vi "Board Measurement.vi"(4 "index":i32, 5 "Board":T1 items=["Quad DC Board", "Lens 1 (Slot 8) Module", "Lens 2 (Slot 6) Module", "Detector Board", "Quad DC Board with Test Points", "Lens 1 Module with Test Points", "Len 2 Module with Test Points", "", "", "", "", ""], 6 "Expected Reading":dbl, 7 "DAC Channel Name":string) -> (1 "Aborted":bool, 3 "Reading":string)   [LabVIEW 2012]
uses:
  Type/_Board ID.ctl
panel:
  in  "AbortButton":bool
  in  "Actual Reading":string
  in  "Done":bool
  # "Please enter an actual reading for the DAC channel below \n(Use the attached picture to locate test points)"
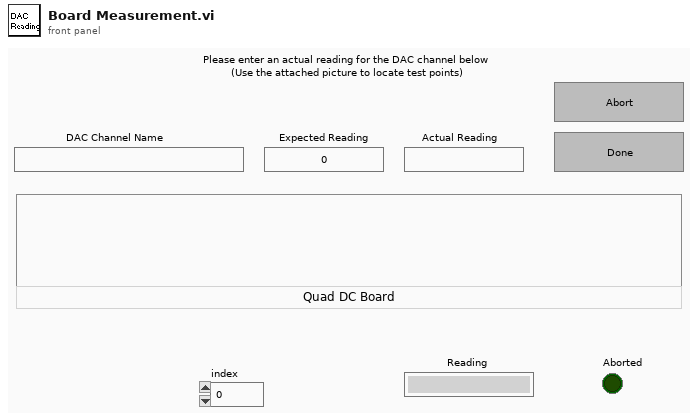
[diagram p1: front panel]
types:
  T1 = typedef "_Board ID.ctl" = u16
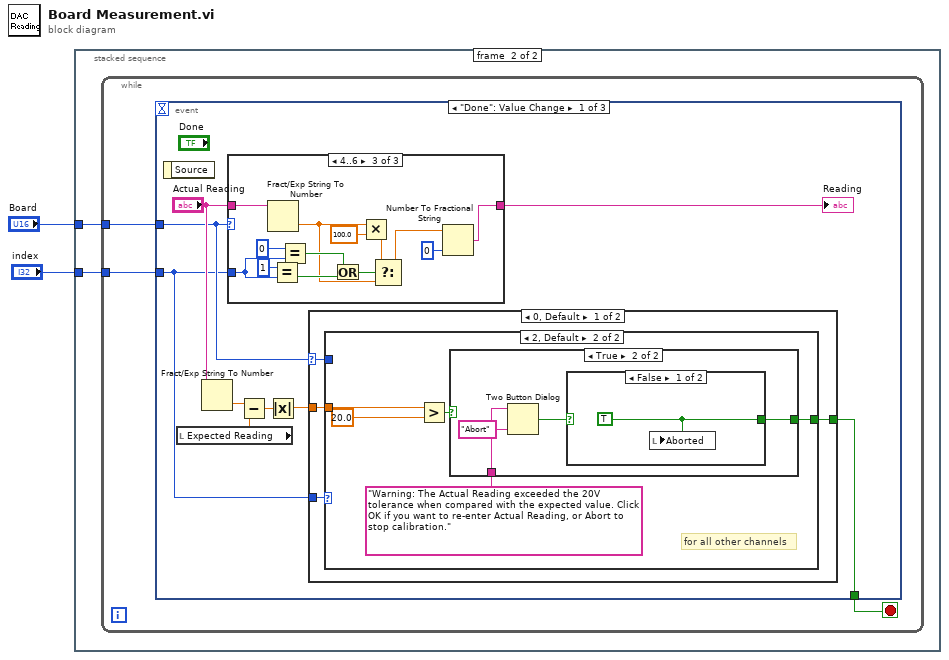
[diagram p0: block diagram]
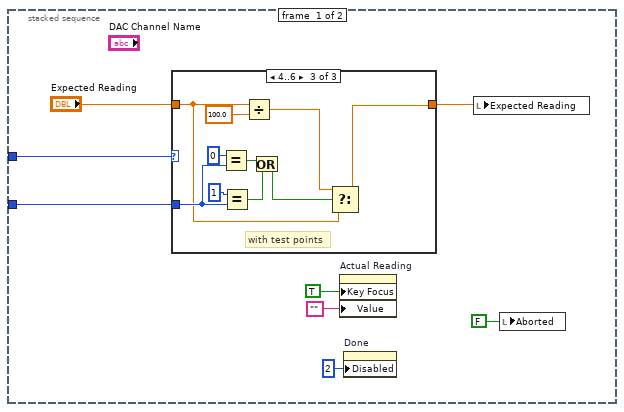
[diagram p2: hidden frame]
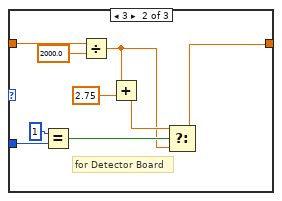
[diagram p4: hidden frame]
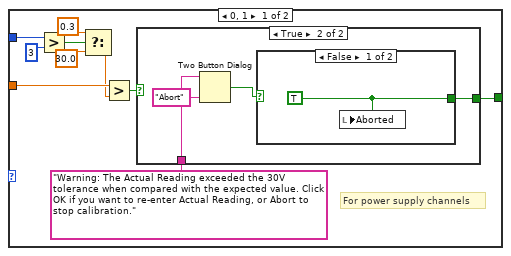
[diagram p5: hidden frame]
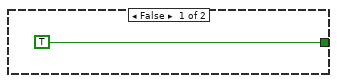
[diagram p6: hidden frame]
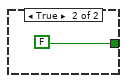
[diagram p7: hidden frame]
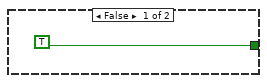
[diagram p8: hidden frame]
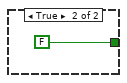
[diagram p9: hidden frame]
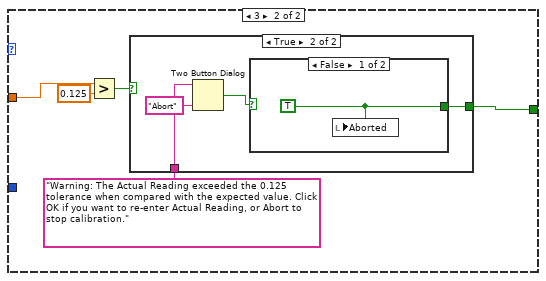
[diagram p10: hidden frame]
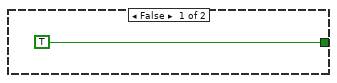
[diagram p11: hidden frame]
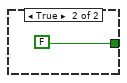
[diagram p12: hidden frame]
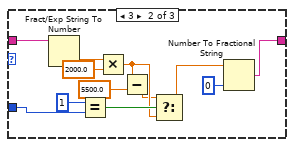
[diagram p14: hidden frame]
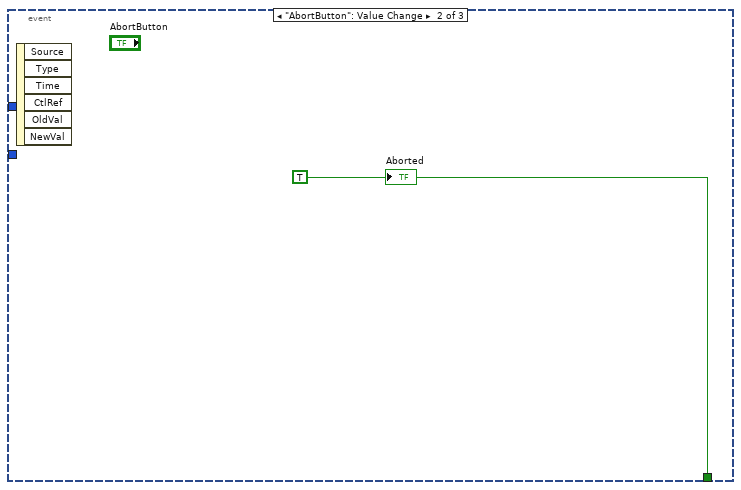
[diagram p15: hidden frame]
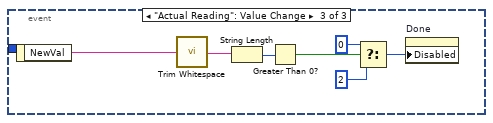
[diagram p16: hidden frame]
diagram:
  n1 = stacked-sequence {
    tunnel: "Board" -> [w7 w32]
    tunnel: "index" -> [w4 w31]
    frame #0 {
      n2 = case shown="4..6" w7 {
        tunnel: "Expected Reading" -> [w11 w20 w21]
        tunnel: [w11 w15 w29] -> w5
        tunnel: w4 -> [_ w18 w26]
        frame 0, Default {
          # "without test points"
        }
        frame 3 {
          # "for Detector Board"
          n3 = Equal?(x=1, y=w18) -> (x = y?=w17:bool)
          n4 = Divide(x=w20, y=2000.0) -> (x/y=w12:dbl)
          n5 = Add(x=w12, y=2.75) -> (x+y=w13:dbl)
          n6 = Select(t=w13, s=w17, f=w12) -> (s? t:f=w15:dbl)
        }
        frame 4..6 {
          # "with test points"
          n7 = Equal?(x=0, y=w26) -> (x = y?=w25:bool)
          n8 = Equal?(x=1, y=w26) -> (x = y?=w24:bool)
          n9 = Divide(x=w21, y=100.0) -> (x/y=w22:dbl)
          n10 = Or(x=w25, y=w24) -> (x .or. y?=w23:bool)
          n11 = Select(t=w22, s=w23, f=w21) -> (s? t:f=w29:dbl)
        }
      }
      n12 = property on="Actual Reading" class="Str"("Key Focus"=TRUE, "Value"="") -> ()  [unwired: 2 in, 2 out]
      n13 = property on="Done" class="Bool"("Disabled"=u8 2) -> ()  [unwired: 2 in, 2 out]
      n14 = local write "Expected Reading"(w5) -> ()
      n15 = local write "Aborted"(FALSE ("Aborted")) -> ()
    }
    frame #1 {
      n16 = while {
        tunnel: w32 -> [w34]
        tunnel: w31 -> [w33]
        stop <- w35 stop-if-true
        n17 = event shown="[0] \"Done\": Value Change" {
          selector: _ -> [_ _ _]
          dyn-events: _ -> [_ _ _]
          timeout: _ -> [_ _ _]
          tunnel: [w38 w116 _] -> w35
          tunnel: w34 -> [w37 _ _]
          tunnel: w33 -> [w36 _ _]
          event "Done": Value Change {
            n18 = event-data() -> ()  [unwired: 2 out]
            n19 = local read "Expected Reading"() -> (w41:dbl)
            n20 = Fract/Exp String To Number(string="Actual Reading") -> (number=w42:dbl)  [unwired: 4 out]
            n21 = case shown="4..6" w37 {
              tunnel: [w90 w98 w112] -> w44
              tunnel: "Actual Reading" -> [w90 w102 w115]
              tunnel: w36 -> [_ w96 w108]
              frame 0, Default {
              }
              frame 3 {
                n22 = Fract/Exp String To Number(string=w102) -> (number=w101:dbl)  [unwired: 4 out]
                n23 = Equal?(x=1, y=w96) -> (x = y?=w97:bool)
                n24 = Multiply(x=w101, y=2000.0) -> (x*y=w92:dbl)
                n25 = Subtract(x=w92, y=5500.0) -> (x-y=w91:dbl)
                n26 = Select(t=w91, s=w97, f=w92) -> (s? t:f=w94:dbl)
                n27 = Number To Fractional String(number=w94, precision (6)=i16 0) -> (F-format string=w98:string)  [unwired: 2 out]
              }
              frame 4..6 {
                n28 = Fract/Exp String To Number(string=w115) -> (number=w103:dbl)  [unwired: 4 out]
                n29 = Equal?(x=1, y=w108) -> (x = y?=w105:bool)
                n30 = Equal?(x=0, y=w108) -> (x = y?=w106:bool)
                n31 = Or(x=w106, y=w105) -> (x .or. y?=w107:bool)
                n32 = Multiply(x=w103, y=100.0) -> (x*y=w104:dbl)
                n33 = Select(t=w104, s=w107, f=w103) -> (s? t:f=w111:dbl)
                n34 = Number To Fractional String(number=w111, precision (6)=i16 0) -> (F-format string=w112:string)  [unwired: 2 out]
              }
            }
            "Reading" <- w44
            n35 = Subtract(x=w42, y=w41) -> (x-y=w40:dbl)
            n36 = Absolute Value(x=w40) -> (abs(x)=w39:dbl)
            n37 = case shown="0, Default" w37 {
              selector: w37 -> [w45 _]
              tunnel: w39 -> [w48 w79]
              tunnel: [w47 w78] -> w38
              tunnel: w36 -> [w46 _]
              frame 0, Default {
                n38 = case shown="2, Default" w46 {
                  tunnel: w48 -> [w51 w70]
                  tunnel: [w49 w68] -> w47
                  tunnel: w45 -> [w58 _]
                  frame 0, 1 {
                    # "For power supply channels"
                    n39 = Greater?(x=w58, y=3) -> (0:w56:bool)
                    n40 = Select(t=0.3 ("y"), s=w56, f=30.0 ("y")) -> (s? t:f=w50:dbl)
                    n41 = Greater?(x=w51, y=w50) -> (0:w53:bool)
                    n42 = case shown="True" w53 {
                      tunnel: [TRUE w60] -> w49
                      tunnel: "Warning: The Actual Reading exceeded the 30V tolerance when compared with the expected value. Click OK if you want to re-enter Actual Reading, or Abort to stop calibration." -> [_ w63]
                      frame False {
                      }
                      frame True {
                        n43 = Two Button Dialog(message=w63, 1:"Abort" ("F button name (\"Cancel\")")) -> (T button?=w61:bool)  [unwired: 1 out]
                        n44 = case shown="False" w61 {
                          tunnel: [w64 FALSE] -> w60
                          frame False {
                            w64 = TRUE
                            n45 = local write "Aborted"(w64) -> ()
                          }
                          frame True {
                          }
                        }
                      }
                    }
                  }
                  frame 2, Default {
                    # "for all other channels"
                    n46 = Greater?(x=w70, y=20.0) -> (0:w69:bool)
                    n47 = case shown="True" w69 {
                      tunnel: [TRUE w73] -> w68
                      tunnel: "Warning: The Actual Reading exceeded the 20V tolerance when compared with the expected value. Click OK if you want to re-enter Actual Reading, or Abort to stop calibration." -> [_ w75]
                      frame False {
                      }
                      frame True {
                        n48 = Two Button Dialog(message=w75, 1:"Abort" ("F button name (\"Cancel\")")) -> (T button?=w74:bool)  [unwired: 1 out]
                        n49 = case shown="False" w74 {
                          tunnel: [w76 FALSE] -> w73
                          frame False {
                            w76 = TRUE
                            n50 = local write "Aborted"(w76) -> ()
                          }
                          frame True {
                          }
                        }
                      }
                    }
                  }
                }
              }
              frame 3 {
                n51 = Greater?(x=w79, y=0.125) -> (0:w81:bool)
                n52 = case shown="True" w81 {
                  tunnel: [TRUE w84] -> w78
                  tunnel: "Warning: The Actual Reading exceeded the 0.125 tolerance when compared with the expected value. Click OK if you want to re-enter Actual Reading, or Abort to stop calibration." -> [_ w87]
                  frame False {
                  }
                  frame True {
                    n53 = Two Button Dialog(message=w87, 1:"Abort" ("F button name (\"Cancel\")")) -> (T button?=w85:bool)  [unwired: 1 out]
                    n54 = case shown="False" w85 {
                      tunnel: [w88 FALSE] -> w84
                      frame False {
                        w88 = TRUE
                        n55 = local write "Aborted"(w88) -> ()
                      }
                      frame True {
                      }
                    }
                  }
                }
              }
            }
          }
          event "AbortButton": Value Change {
            w116 = TRUE ("Aborted")
            n56 = event-data() -> ()  [unwired: 7 out]
            "Aborted" <- w116
          }
          event "Actual Reading": Value Change {
            n57 = event-data() -> ("NewVal"=w118:string)  [unwired: 1 out]
            n58 = call <vilib>:"Trim Whitespace.vi"("string"=w118) -> ("trimmed string"=w123:string)  [unwired: 1 in]
            n59 = String Length(string=w123) -> (length=w122:i32)
            n60 = Greater Than 0?(x=w122) -> (x > 0?=w117:bool)
            n61 = Select(t=u8 0, s=w117, f=u8 2 ("Disabled")) -> (s? t:f=w119:u8)
            n62 = property on="Done" class="Bool"("Disabled"=w119) -> ()  [unwired: 2 in, 2 out]
          }
        }
      }
    }
  }
